vi "Teleop - Hood Angle Adjustment (SubVI).vi"(0 "turretAngleDesired In":dbl, 1 "kickupWheelDesired In":dbl, 2 "hoodAngleDesired In":dbl, 3 "sideConveyorDesired In":dbl, 4 "Constant Cluster In":T1 {"12. Auton Deriv Drive Straight Gain" format="%_6f"; "11. Auton Int Drive Straight Gain" format="%_6f"; "10. Auton Prop Drive Straight Gain" format="%_6f"; "9. Auton I Output Limit Turn Gain" format="%_6f"; "8. Auton Deriv Turn Gain" format="%_6f"; "7. Auton Int Turn Gain" format="%_6f"; "1. Auton Prop Drive Gain" format="%_6f"; "2. Auton Int Drive Gain" format="%_6f"; "3. Auton Deriv Drive Gain" format="%_6f"; "4. I Output Drive  Limit" format="%_6f"; "5. Auto Drive Cheat (%)" format="%_6f"; "6. Auton Prop Turn Gain" format="%_6f"}, 5 "shooterVelocityActual":dbl) -> (14 "turretAngleDesired Out":dbl, 15 "kickupWheelDesired Out":dbl, 16 "hoodAngleDesired Out":dbl, 17 "sideConveyorDesired Out":dbl, 18 "Constant Cluster Out":T1 {"12. Auton Deriv Drive Straight Gain" format="%_6f"; "11. Auton Int Drive Straight Gain" format="%_6f"; "10. Auton Prop Drive Straight Gain" format="%_6f"; "9. Auton I Output Limit Turn Gain" format="%_6f"; "8. Auton Deriv Turn Gain" format="%_6f"; "7. Auton Int Turn Gain" format="%_6f"; "1. Auton Prop Drive Gain" format="%_6f"; "2. Auton Int Drive Gain" format="%_6f"; "3. Auton Deriv Drive Gain" format="%_6f"; "4. I Output Drive  Limit" format="%_6f"; "5. Auto Drive Cheat (%)" format="%_6f"; "6. Auton Prop Turn Gain" format="%_6f"})   [LabVIEW 2019]
uses:
  Disabled/Constant VI_s/Disabled - Constant Cluster Typedef.ctl
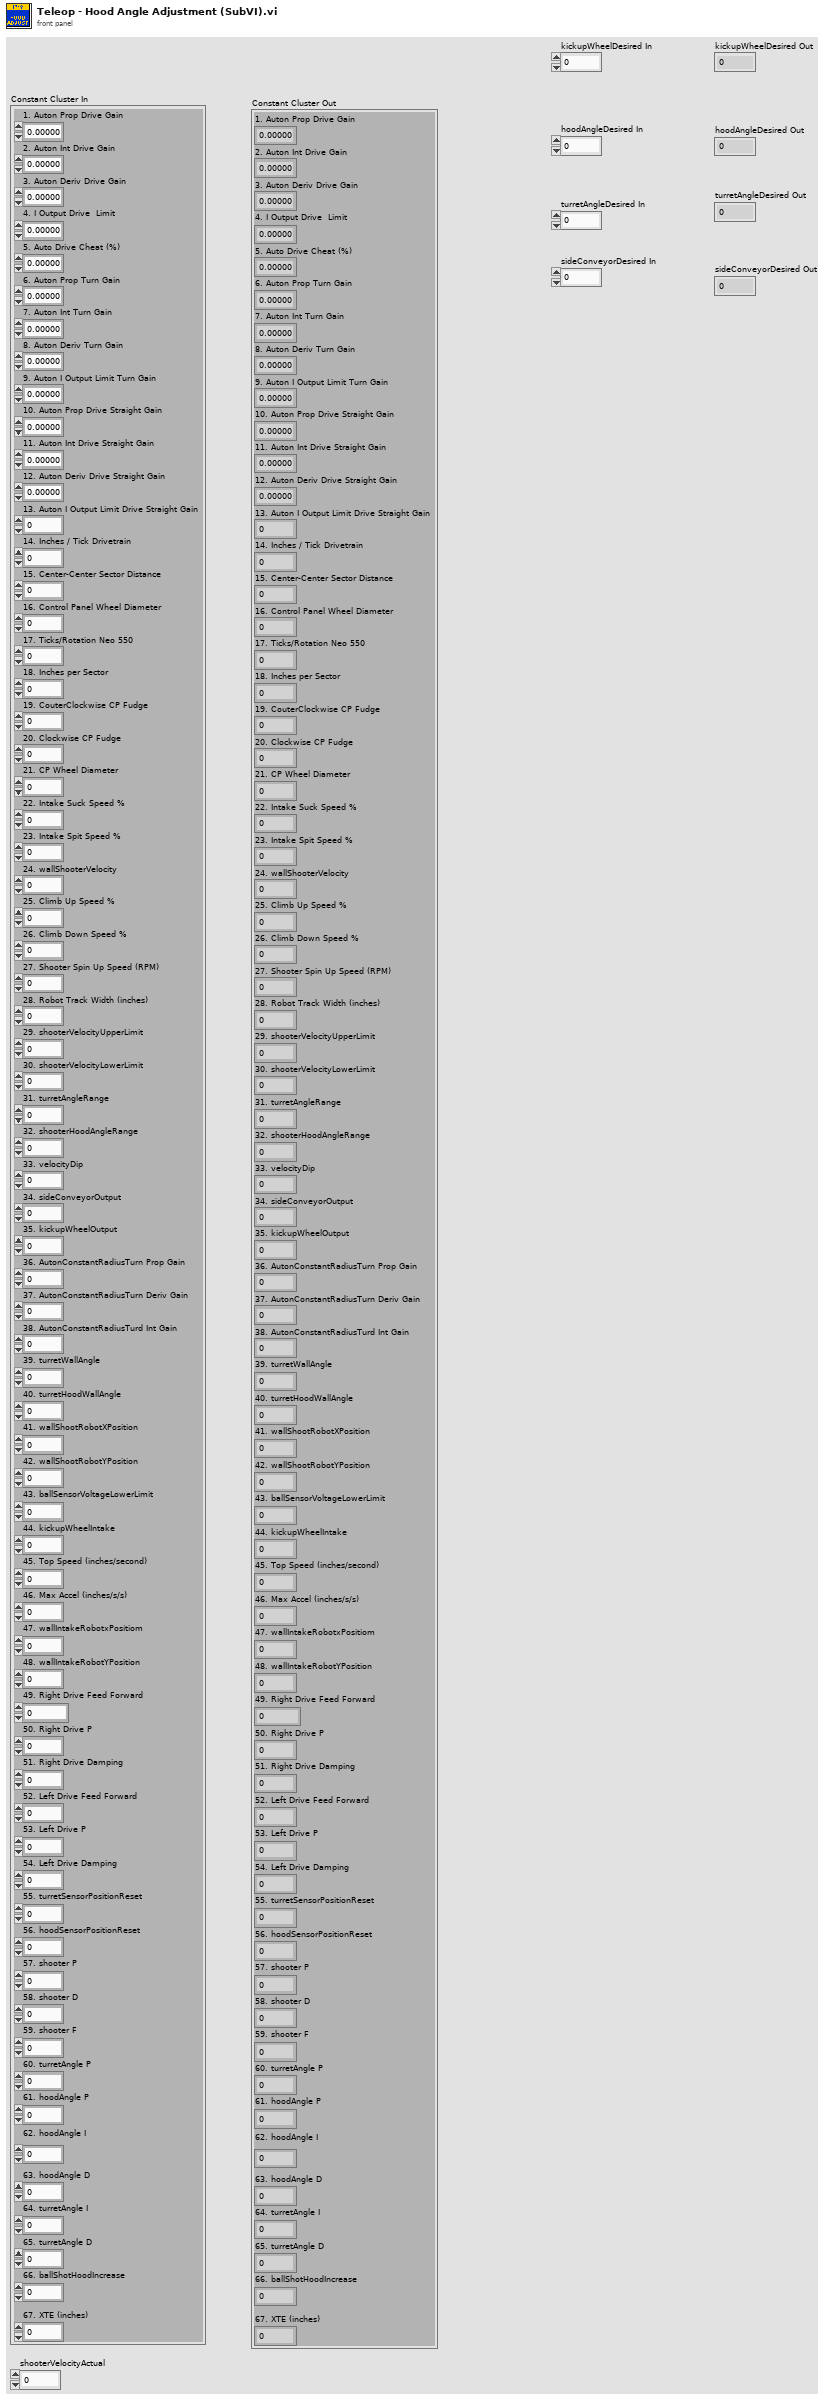
[diagram p1: front panel]
types:
  T1 = typedef "Disabled - Constant Cluster Typedef.ctl" = cluster{"1. Auton Prop Drive Gain":dbl, "2. Auton Int Drive Gain":dbl, "3. Auton Deriv Drive Gain":dbl, "4. I Output Drive  Limit":dbl, "5. Auto Drive Cheat (%)":dbl, "6. Auton Prop Turn Gain":dbl, "7. Auton Int Turn Gain":dbl, "8. Auton Deriv Turn Gain":dbl, "9. Auton I Output Limit Turn Gain":dbl, "10. Auton Prop Drive Straight Gain":dbl, "11. Auton Int Drive Straight Gain":dbl, "12. Auton Deriv Drive Straight Gain":dbl, "13. Auton I Output Limit Drive Straight Gain":dbl, "14. Inches / Tick Drivetrain":dbl, "15. Center-Center Sector Distance":dbl, "16. Control Panel Wheel Diameter":dbl, "17. Ticks/Rotation Neo 550":dbl, "18. Inches per Sector":dbl, "19. CouterClockwise CP Fudge":dbl, "20. Clockwise CP Fudge":dbl, "21. CP Wheel Diameter":dbl, "22. Intake Suck Speed %":dbl, "23. Intake Spit Speed %":dbl, "24. wallShooterVelocity":dbl, "25. Climb Up Speed %":dbl, "26. Climb Down Speed %":dbl, "27. Shooter Spin Up Speed (RPM)":dbl, "28. Robot Track Width (inches)":dbl, "29. shooterVelocityUpperLimit":dbl, "30. shooterVelocityLowerLimit":dbl, "31. turretAngleRange":dbl, "32. shooterHoodAngleRange":dbl, "33. velocityDip":dbl, "34. sideConveyorOutput":dbl, "35. kickupWheelOutput":dbl, "36. AutonConstantRadiusTurn Prop Gain":dbl, "37. AutonConstantRadiusTurn Deriv Gain":dbl, "38. AutonConstantRadiusTurd Int Gain":dbl, "39. turretWallAngle":dbl, "40. turretHoodWallAngle":dbl, "41. wallShootRobotXPosition":dbl, "42. wallShootRobotYPosition":dbl, "43. ballSensorVoltageLowerLimit":dbl, "44. kickupWheelIntake":dbl, "45. Top Speed (inches/second)":dbl, "46. Max Accel (inches/s/s)":dbl, "47. wallIntakeRobotxPositiom":dbl, "48. wallIntakeRobotYPosition":dbl, "49. Right Drive Feed Forward":dbl, "50. Right Drive P":dbl, "51. Right Drive Damping":dbl, "52. Left Drive Feed Forward":dbl, "53. Left Drive P":dbl, "54. Left Drive Damping":dbl, "55. turretSensorPositionReset":dbl, "56. hoodSensorPositionReset":dbl, "57. shooter P":dbl, "58. shooter D":dbl, "59. shooter F":dbl, "60. turretAngle P":dbl, "61. hoodAngle P":dbl, "62. hoodAngle I":dbl, "63. hoodAngle D":dbl, "64. turretAngle I":dbl, "65. turretAngle D":dbl, "66. ballShotHoodIncrease":dbl, "67. XTE (inches)":dbl}
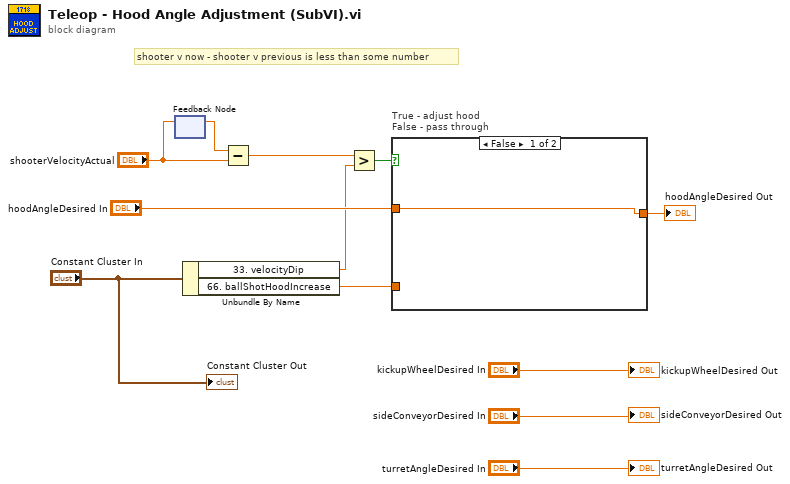
[diagram p0: block diagram]
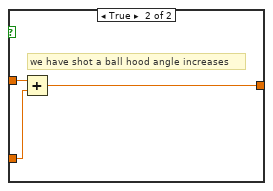
[diagram p2: hidden frame]
diagram:
  # "shooter v now - shooter v previous is less than some number"
  n1 = feedback #1() -> (w8:dbl)  [unwired: 1 in]
  n2 = feedback-in #1("shooterVelocityActual") -> ()
  n3 = Unbundle By Name("Constant Cluster In") -> ("33. velocityDip"=w6:dbl, "66. ballShotHoodIncrease"=w12:dbl)
  n4 = Subtract(x=w8, y="shooterVelocityActual") -> (x-y=w5:dbl)
  n5 = Greater?(x=w5, y=w6) -> (0:w7:bool)
  n6 = case "True - adjust hood \nFalse - pass through" shown="False" w7 {
    tunnel: [w13 w15] -> w10
    tunnel: "hoodAngleDesired In" -> [w13 w16]
    tunnel: w12 -> [_ w14]
    frame False {
    }
    frame True {
      # "we have shot a ball hood angle increases"
      n7 = Add(x=w16, y=w14) -> (x+y=w15:dbl)
    }
  }
  "hoodAngleDesired Out" <- w10
  "kickupWheelDesired Out" <- "kickupWheelDesired In"
  "sideConveyorDesired Out" <- "sideConveyorDesired In"
  "turretAngleDesired Out" <- "turretAngleDesired In"
  "Constant Cluster Out" <- "Constant Cluster In"
